vi "serial_facade.vi"(0 "Data In":T4, 2 "Display State In":T2, 3 "Container State":T3) -> (6 "Data Out":T4, 7 "Display State Out":T2, 8 "Action":T1)   [LabVIEW 2022 SP3, in "Serial_Port.xctl"]
uses:
  Serial_Port.xctl
  serial_data.ctl
  Processors.ctl
  <vilib>/_xctls/Container State.ctl
  serial_state.ctl
  <vilib>/_xctls/Action.ctl
  <vilib>/_xctls/XControlSupport.lvlib
panel:
  in  "refresh":bool
  in  "Port":string(combo)
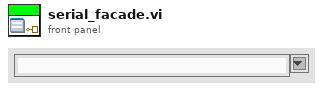
[diagram p1: front panel]
types:
  T1 = typedef "XControlSupport.lvlib/Action.ctl" = cluster{"Data Changed?":bool, "State Changed?":bool, "Action Name":string}
  T2 = typedef "Serial_Port.xctl/serial_state.ctl" = cluster{"Numeric":dbl}
  T3 = typedef "XControlSupport.lvlib/Container State.ctl" = cluster{"Indicator?":bool, "Run Mode?":bool, " Refnum":refnum<vi>}
  T4 = typedef "Serial_Port.xctl/serial_data.ctl" = cluster{"session":refnum<k35>, "PyPath":path, "Processor":T5, "Port":string, "version":string}
  T5 = typedef "Processors.ctl" = enum16{"SPIKE", "Pi", "Pi_ssh", "OpenMV", "Dunio"}
  T6 = typedef "Preferences.ctl" = cluster{"python":string, "arduino CLI":path, "pythonCodes":cluster{"pythonCode":path, "Color":u32}[], "FontSize":u8, "Text Colors":cluster{"Quote":u32, "function":u32, "Python":u32, "Comment":u32, "Triple Quote":u32, "Text":u32}, "SSH Logins":cluster{"IP Address":string, "Username":string, "password":string}[], "packet size":u8}
  T7 = typedef "PythonCtrl.ctl" = cluster{"session":refnum<k35>, "PyPath":path, "Processor":T5, "Port":string, "version":string}
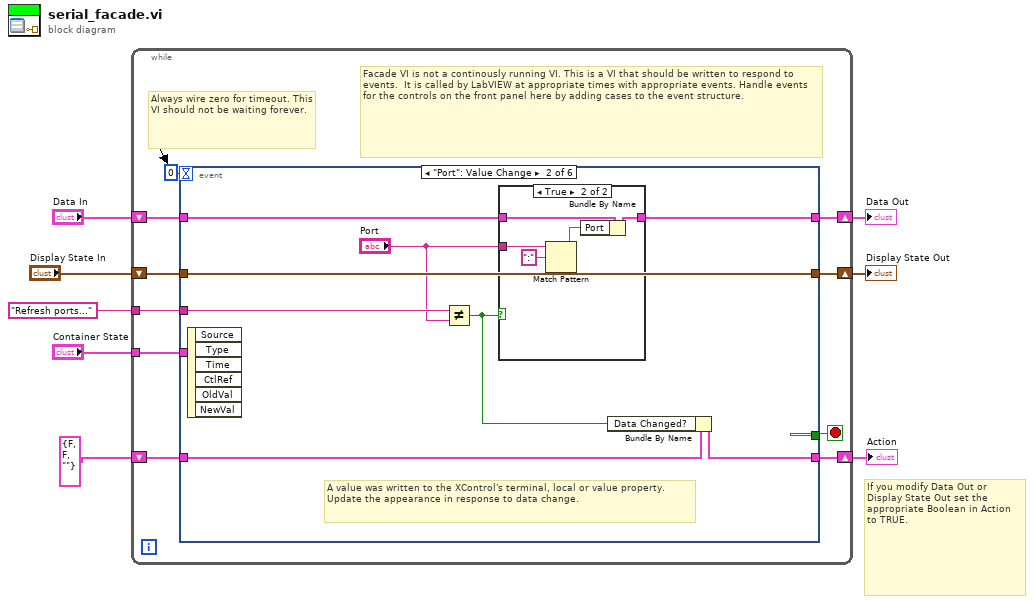
[diagram p0: block diagram]
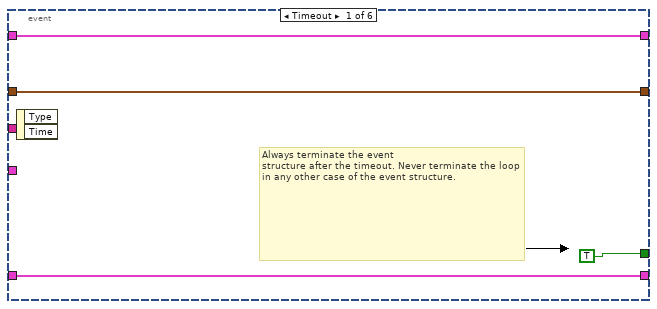
[diagram p2: hidden frame]
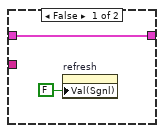
[diagram p3: hidden frame]
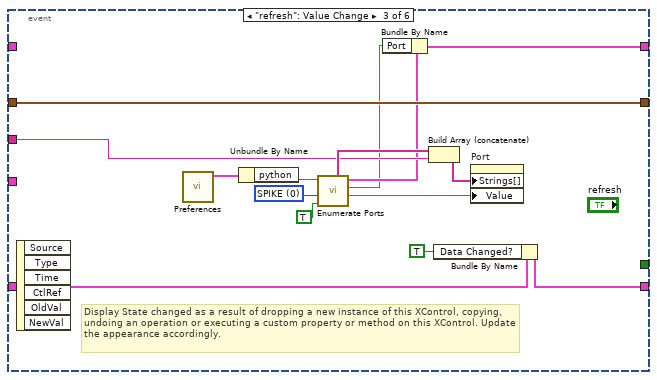
[diagram p4: hidden frame]
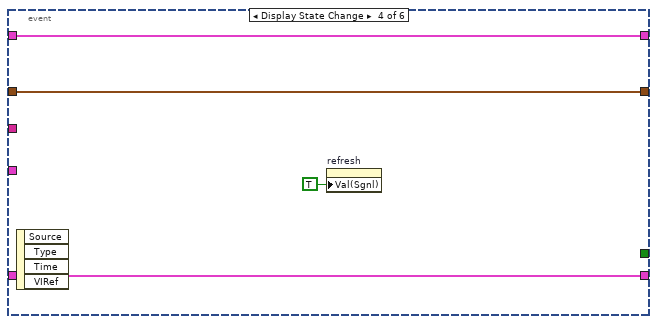
[diagram p5: hidden frame]
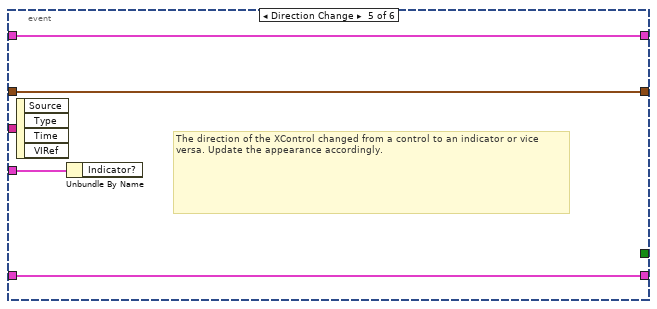
[diagram p6: hidden frame]
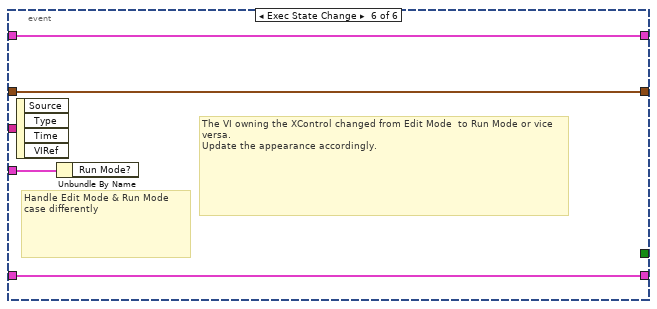
[diagram p7: hidden frame]
diagram:
  # "If you modify Data Out or\nDisplay State Out set the\nappropriate Boolean in Action\nto TRUE."
  n1 = while {
    shift-right: [w17] -> w5
    shift-left: "Display State In" -> [w18]
    tunnel: "Container State" -> [w14]
    shift-right: [w12] -> w8
    shift-left: "Data In" -> [w13]
    shift-right: [w10] -> w3
    shift-left: T1 {"Data Changed?"=FALSE, "State Changed?"=FALSE, "Action Name"=""} ("Action") -> [w11]
    tunnel: "Refresh ports..." -> [w9]
    stop <- w16 stop-if-true
    # "Facade VI is not a continously running VI. This is a VI that should be written to respond to events.  It is called by LabVIEW at appropriate times with appropriate events. Handle events for the controls on the front panel here by adding cases to the event structure."
    # "Always wire zero for timeout. This\nVI should not be waiting forever."
    n2 = event shown="[1] \"Port\": Value Change" {
      selector: _ -> [_ _ _ _ _ _]
      dyn-events: _ -> [_ _ _ _ _ _]
      timeout: 0 -> [_ _ _ _ _ _]
      tunnel: w18 -> [w20 w30 w52 w56 w59 w63]
      tunnel: [w20 w30 w52 w56 w59 w63] -> w17
      tunnel: [TRUE _ _ _ _ _] -> w16
      tunnel: w14 -> [_ _ _ _ w60 w64]
      tunnel: w13 -> [w19 w25 _ w55 w58 w62]
      tunnel: [w19 w27 w38 w55 w58 w62] -> w12
      tunnel: [w21 w29 w46 w54 w57 w61] -> w10
      tunnel: w11 -> [w21 w28 w45 w54 w57 w61]
      tunnel: w9 -> [_ w26 w41 _ _ _]
      event Timeout {
        # "Always terminate the event\nstructure after the timeout. Never terminate the loop in any other case of the event structure."
        n3 = event-data() -> ()  [unwired: 1 in, 2 out]
      }
      event "Port": Value Change {
        # "A value was written to the XControl's terminal, local or value property.\nUpdate the appearance in response to data change."
        n4 = event-data() -> ()  [unwired: 1 in, 6 out]
        n5 = Not Equal?(x=w26, y="Port") -> (x != y?=w24:bool)
        n6 = case shown="True" w24 {
          tunnel: [w32 w34] -> w27
          tunnel: "Port" -> [_ w36]
          tunnel: w25 -> [w32 w35]
          frame False {
            n7 = property on="refresh" class="Bool (strict)"("Val(Sgnl)"=FALSE ("Value (Signaling)")) -> ()  [unwired: 2 in, 2 out]
          }
          frame True {
            n8 = Match Pattern(string=w36, regular expression=":") -> (before substring=w33:string)  [unwired: 1 in, 3 out]
            n9 = Bundle By Name(cluster=w35, "Port"=w33) -> (w34:T4)
          }
        }
        n10 = Bundle By Name(cluster=w28, "Data Changed?"=w24) -> (w29:T1)
      }
      event "refresh": Value Change {
        w50 = u16 0 items=["SPIKE", "Pi", "Pi_ssh", "OpenMV", "duino"] ("Processor")
        # "Display State changed as a result of dropping a new instance of this XControl, copying, undoing an operation or executing a custom property or method on this XControl. Update the appearance accordingly."
        n11 = event-data() -> ()  [unwired: 1 in, 6 out]
        n12 = call "Preferences.vi"() -> ("Preferences out"=w51:T6)  [unwired: 10 in, 1 out]
        n13 = Unbundle By Name(w51) -> ("python"=w49:string)
        n14 = call "Enumerate Ports.vi"("list?"=TRUE, "Processor"=w50, "Python version"=w49) -> ("guess"=w47:string, "Short guess"=w39:string, "Python"=w40:T7, "possibilities"=w43:string[])  [unwired: 3 in, 2 out]
        n15 = Bundle By Name(cluster=w40, "Port"=w39) -> (w38:T7)
        n16 = Build Array (concatenate)(w43, w41) -> (w42:string[])
        n17 = Bundle By Name(cluster=w45, "Data Changed?"=TRUE) -> (w46:T1)
        n18 = property on="Port" class="CmbBox"("Strings[]"=w42, "Value"=w47) -> ()  [unwired: 2 in, 2 out]
      }
      event Display State Change {
        n19 = event-data() -> ()  [unwired: 1 in, 4 out]
        n20 = property on="refresh" class="Bool (strict)"("Val(Sgnl)"=TRUE ("Value (Signaling)")) -> ()  [unwired: 2 in, 2 out]
      }
      event Direction Change {
        # "The direction of the XControl changed from a control to an indicator or vice versa. Update the appearance accordingly."
        n21 = event-data() -> ()  [unwired: 1 in, 4 out]
        n22 = Unbundle By Name(w60) -> ()  [unwired: 1 out]
      }
      event Exec State Change {
        # "The VI owning the XControl changed from Edit Mode  to Run Mode or vice versa.\nUpdate the appearance accordingly."
        # "Handle Edit Mode & Run Mode\ncase differently"
        n23 = event-data() -> ()  [unwired: 1 in, 4 out]
        n24 = Unbundle By Name(w64) -> ()  [unwired: 1 out]
      }
    }
  }
  "Display State Out" <- w5
  "Data Out" <- w8
  "Action" <- w3
